vi "DTC Descriptor FG.vi"(7 "Action":T1, 8 "error in (no error)":errorcluster, 10 "DTC descriptor":T2={"DTC Byte Length"=2, "Status Byte Length"=1, "Add Data Byte Length"=1, "Byte Order"=enum."Motorola"}, 11 "Device Item Ref in":T3 format="%.0x") -> (0 "error out":errorcluster, 2 "DTC descriptor":T2={"DTC Byte Length"=2, "Status Byte Length"=1, "Add Data Byte Length"=1, "Byte Order"=enum."Motorola"}, 3 "Device Item Ref out":T3=18446744073709551615 format="%.0x")   [LabVIEW 2015, in "Diagnostics Addon System Explorer.lvlib"]
uses:
  Diagnostics Addon System Explorer.lvlib
  <vilib>/NI Veristand/Custom Device API/Custom Device Item Ref.ctl
  Shared/Types/DTC Descriptor Parameters.ctl
  Types/FG Action.ctl
  <vilib>/NI Veristand/Custom Device API/Get Item Property (U32).vi
  <vilib>/NI Veristand/Custom Device API/Get Item Property (I32).vi
  <vilib>/NI Veristand/Custom Device API/Set Item Property (U32).vi
  <vilib>/NI Veristand/Custom Device API/Set Item Property (I32).vi
  Shared/SubVIs/GUID Lookup.vi
  Shared/Diagnostics Addon Shared.lvlib
  <vilib>/NI Veristand/Custom Device API/Custom Device API.lvlib
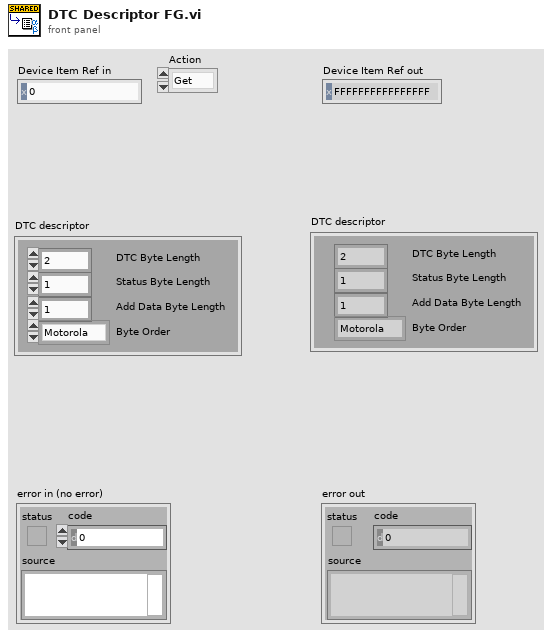
[diagram p1: front panel]
types:
  T1 = typedef "Diagnostics Addon System Explorer.lvlib/FG Action.ctl" = enum16{"Get", "Set"}
  T2 = typedef "Diagnostics Addon Shared.lvlib/DTC Descriptor Parameters.ctl" = cluster{"DTC Byte Length":i32, "Status Byte Length":i32, "Add Data Byte Length":i32, "Byte Order":enum16{"Motorola", "Intel"}}
  T3 = typedef "Custom Device API.lvlib/Custom Device Item Ref.ctl" = u64
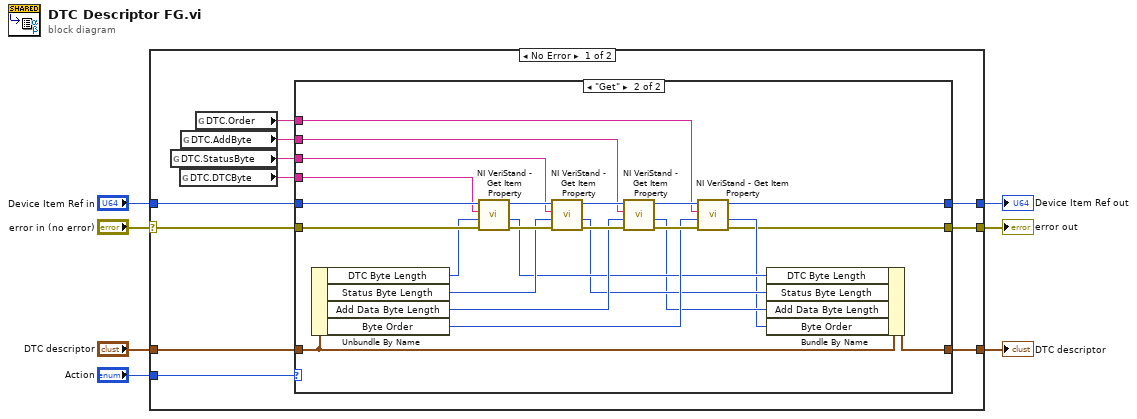
[diagram p0: block diagram]
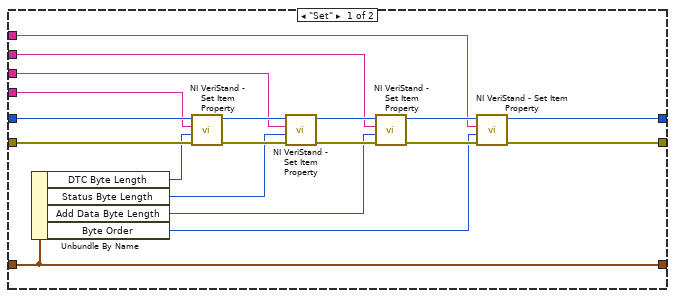
[diagram p2: hidden frame]
diagram:
  n1 = case shown="No Error" "error in (no error)" {
    selector: "error in (no error)" -> [w18 w62]
    tunnel: "Device Item Ref in" -> [w17 w63]
    tunnel: [w16 w63] -> w4
    tunnel: [w15 w62] -> w5
    tunnel: [w14 _] -> w3
    tunnel: "DTC descriptor" -> [w13 _]
    tunnel: "Action" -> [w12 _]
    frame No Error {
      n2 = global read "GUID Lookup.vi" "DTC.StatusByte"() -> (w10:string)
      n3 = global read "GUID Lookup.vi" "DTC.DTCByte"() -> (w11:string)
      n4 = global read "GUID Lookup.vi" "DTC.AddByte"() -> (w9:string)
      n5 = global read "GUID Lookup.vi" "DTC.Order"() -> (w8:string)
      n6 = case shown="\"Get\"" w12 {
        tunnel: w18 -> [w37 w61]
        tunnel: w17 -> [w36 w60]
        tunnel: [w30 w53] -> w16
        tunnel: [w31 w38] -> w15
        tunnel: [w35 w39] -> w14
        tunnel: w13 -> [w35 w44]
        tunnel: w11 -> [w21 w48]
        tunnel: w10 -> [w20 w47]
        tunnel: w9 -> [w19 w46]
        tunnel: w8 -> [w26 w45]
        frame "Set" {
          n7 = Unbundle By Name(w35) -> ("DTC Byte Length"=w22:i32, "Status Byte Length"=w23:i32, "Add Data Byte Length"=w24:i32, "Byte Order"=w25:enum16{"Motorola", "Intel"})
          n8 = call-poly <vilib>:"NI VeriStand - Set Item Property.vi"("error in (no error)"=w37, "Value"=w22, "Property Name"=w21, "Item Ref in"=w36) -> ("error out"=w34:errorcluster, "Item Ref out"=w27:T3)  [unwired: 5 in, 1 out]
          n9 = call-poly <vilib>:"NI VeriStand - Set Item Property.vi"("error in (no error)"=w34, "Value"=w23, "Property Name"=w20, "Item Ref in"=w27) -> ("error out"=w33:errorcluster, "Item Ref out"=w28:T3)  [unwired: 5 in, 1 out]
          n10 = call-poly <vilib>:"NI VeriStand - Set Item Property.vi"("error in (no error)"=w33, "Value"=w24, "Property Name"=w19, "Item Ref in"=w28) -> ("error out"=w32:errorcluster, "Item Ref out"=w29:T3)  [unwired: 5 in, 1 out]
          n11 = call-poly <vilib>:"NI VeriStand - Set Item Property.vi"("error in (no error)"=w32, "Value"=w25, "Property Name"=w26, "Item Ref in"=w29) -> ("error out"=w31:errorcluster, "Item Ref out"=w30:T3)  [unwired: 5 in, 1 out]
        }
        frame "Get" {
          n12 = Unbundle By Name(w44) -> ("DTC Byte Length"=w52:i32, "Status Byte Length"=w51:i32, "Add Data Byte Length"=w50:i32, "Byte Order"=w49:enum16{"Motorola", "Intel"})
          n13 = call-poly <vilib>:"NI VeriStand - Get Item Property.vi"("error in (no error)"=w61, "Default Value"=w52, "Property Name"=w48, "Item Ref in"=w60) -> ("error out"=w59:errorcluster, "Value"=w43:i32, "Item Ref out"=w56:T3)  [unwired: 4 in, 1 out]
          n14 = call-poly <vilib>:"NI VeriStand - Get Item Property.vi"("error in (no error)"=w59, "Default Value"=w51, "Property Name"=w47, "Item Ref in"=w56) -> ("error out"=w58:errorcluster, "Value"=w42:i32, "Item Ref out"=w55:T3)  [unwired: 4 in, 1 out]
          n15 = call-poly <vilib>:"NI VeriStand - Get Item Property.vi"("error in (no error)"=w58, "Default Value"=w50, "Property Name"=w46, "Item Ref in"=w55) -> ("error out"=w57:errorcluster, "Value"=w41:i32, "Item Ref out"=w54:T3)  [unwired: 4 in, 1 out]
          n16 = call-poly <vilib>:"NI VeriStand - Get Item Property.vi"("error in (no error)"=w57, "Default Value"=w49, "Property Name"=w45, "Item Ref in"=w54) -> ("error out"=w38:errorcluster, "Value"=w40:u32, "Item Ref out"=w53:T3)  [unwired: 4 in, 1 out]
          n17 = Bundle By Name(cluster=w44, "DTC Byte Length"=w43, "Status Byte Length"=w42, "Add Data Byte Length"=w41, "Byte Order"=w40) -> (w39:T2)
        }
      }
    }
    frame Error {
    }
  }
  "error out" <- w5
  "Device Item Ref out" <- w4
  "DTC descriptor" <- w3
